vi "test.vi"() -> ()   [LabVIEW 2010, in "ErrorController.lvclass"]
uses:
  ErrorController.lvclass
  class_data.vi
panel:
  in  "source":string="123"
  out "error out 2":errorcluster
  out "error out":errorcluster
  out "initialization succesful loaded?":bool
  in  "additional message":string="Test message in test.vi"
  in  "error file store path":path
  in  "send error":bool
  in  "stop":bool
  # "Specify the error file store path before running this VI!!!"
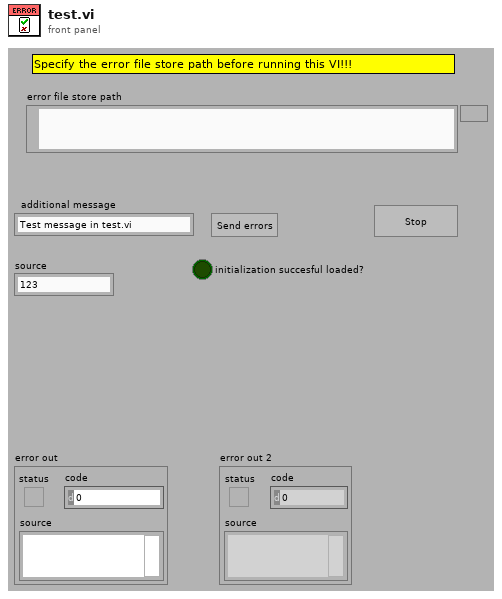
[diagram p1: front panel]
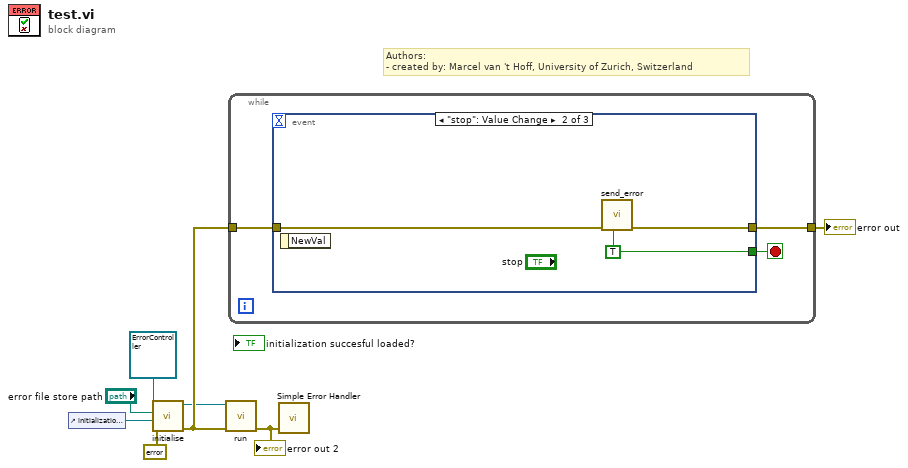
[diagram p0: block diagram]
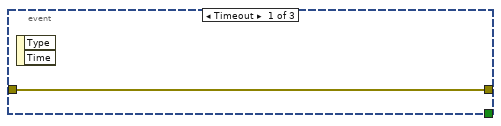
[diagram p2: hidden frame]
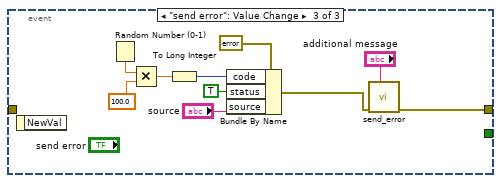
[diagram p3: hidden frame]
diagram:
  # "Authors: \n- created by: Marcel van 't Hoff, University of Zurich, Switzerland"
  n1 = control-ref of="initialization succesful loaded?"() -> (w2:refnum<vi>)
  n2 = call-dynamic "initialise.vi"("error in (no error)"=errorcluster {"status"=FALSE, "code"=0, "source"=""} ("error IO"), "error boolean"=w2, "error file store path"="error file store path", "ErrorController in"=refnum<class "ErrorController.lvclass"> refnum ("ErrorControllerMH101102 in")) -> ("error out"=w6:errorcluster, "ErrorController out"=w3:refnum<class "ErrorController.lvclass">)  [unwired: 6 in]
  n3 = call "run.vi"("error in (no error)"=w6, "ErrorController in"=w3) -> ("error out"=w8:errorcluster)  [unwired: 8 in, 1 out]
  "error out 2" <- w8
  n4 = while {
    tunnel: w6 -> [w11]
    tunnel: [w10] -> w1
    stop <- w9 stop-if-true
    n5 = event shown="[1] \"stop\": Value Change" {
      selector: _ -> [_ _ _]
      dyn-events: _ -> [_ _ _]
      timeout: _ -> [_ _ _]
      tunnel: w11 -> [w12 w15 _]
      tunnel: [w12 w14 w25] -> w10
      tunnel: [_ w13 _] -> w9
      event Timeout {
        n6 = event-data() -> ()  [unwired: 1 in, 2 out]
      }
      event "stop": Value Change {
        w13 = TRUE ("force submission? (F)")
        n7 = event-data() -> ()  [unwired: 1 in, 1 out]
        n8 = call "send_error.vi"("last error? (F)"=w13, "error in (no error)"=w15) -> ("error out"=w14:errorcluster)  [unwired: 9 in]
      }
      event "send error": Value Change {
        n9 = event-data() -> ()  [unwired: 1 in, 1 out]
        n10 = Random Number (0-1)() -> (number: 0 to 1=w22:dbl)
        n11 = Multiply(x=w22, y=100.0) -> (x*y=w20:dbl)
        n12 = To Long Integer(number=w20) -> (32bit integer=w19:i32)
        n13 = Bundle By Name(cluster=errorcluster {"status"=FALSE, "code"=0, "source"=""} ("error out"), "code"=w19, "status"=TRUE, "source"="source") -> (w18:errorcluster)
        n14 = call "send_error.vi"("additional message"="additional message", "error in (no error)"=w18) -> ("error out"=w25:errorcluster)  [unwired: 9 in]
      }
    }
  }
  "error out" <- w1
  n15 = call <vilib>:"Simple Error Handler.vi"("error in (no error)"=w8) -> ()  [unwired: 4 in, 5 out]
